vi "Word Report - Generate from Template.vi"() -> ()   [LabVIEW 2023]
doc: "This example shows how to generate a report from a Word document template. The template contains a preformatted table and a preformatted graph which are updated with Append Table to Report.vi and Excel Update Graph.vi."
uses:
  <vilib>/Utility/NIReport.llb/Report Type.ctl
  <vilib>/Utility/NIReport.llb/Append Report Text (str wrap).vi
  <vilib>/addons/_office/word.llb/Word Edit Cell ([str]).vi
  <vilib>/Utility/NIReport.llb/NI_report.lvclass
  <vilib>/addons/_office/NI_ReportGenerationToolkit.lvlib
  <vilib>/Utility/NIReport.llb/Word/NI_Word.lvclass
  <vilib>/Utility/NIReport.llb/NI_ReportGenerationCore.lvlib
panel:
  in  "Express VI?":bool
  in  "Test operator":string="Operator's name"
  in  "Pressure":string="100"
  in  "Humidity":string="70"
  in  "Temperature":string="20"
  in  "Data":string[][](table)=[["100", "41.7", "38.5"], ["125", "41.7", "35.2"], ["160", "41.5", "37.5"], ["200", "42.3", "42.5"], ["250", "46.9", "46.8"], ["315", "51.9", "52.6"], ["400", "52.3", "46.7"], ["500  ", "46.5", "41.6"], ["630", "42.3", "35.9"], ["800", "41.1", "32.6"]]
  # "Overview: This example shows how to generate a report from a template using either \nthe Word Report Generation VIs or the MS Office Report Express VI.\nRequirements: Report Generation Toolkit, Microsoft Word\nInstructions:\nRun the VI."
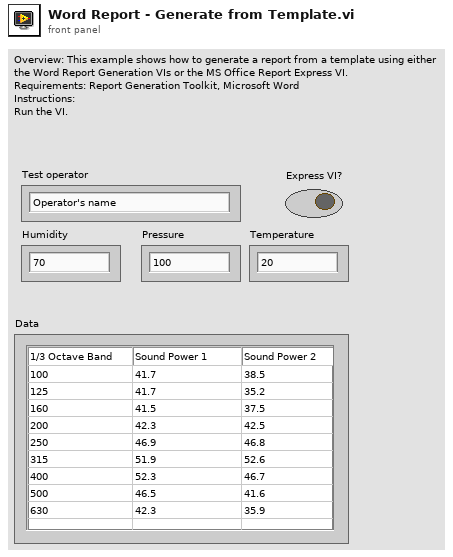
[diagram p1: front panel]
types:
  T1 = typedef "NI_ReportGenerationCore.lvlib/Report Type.ctl" = enum16{"HTML", "Word", "Excel"}
  T2 = cluster{"position (Excel)":cluster{"row":i32, "column":i32}, "name (Excel)":string, "bookmark (Word)":string}
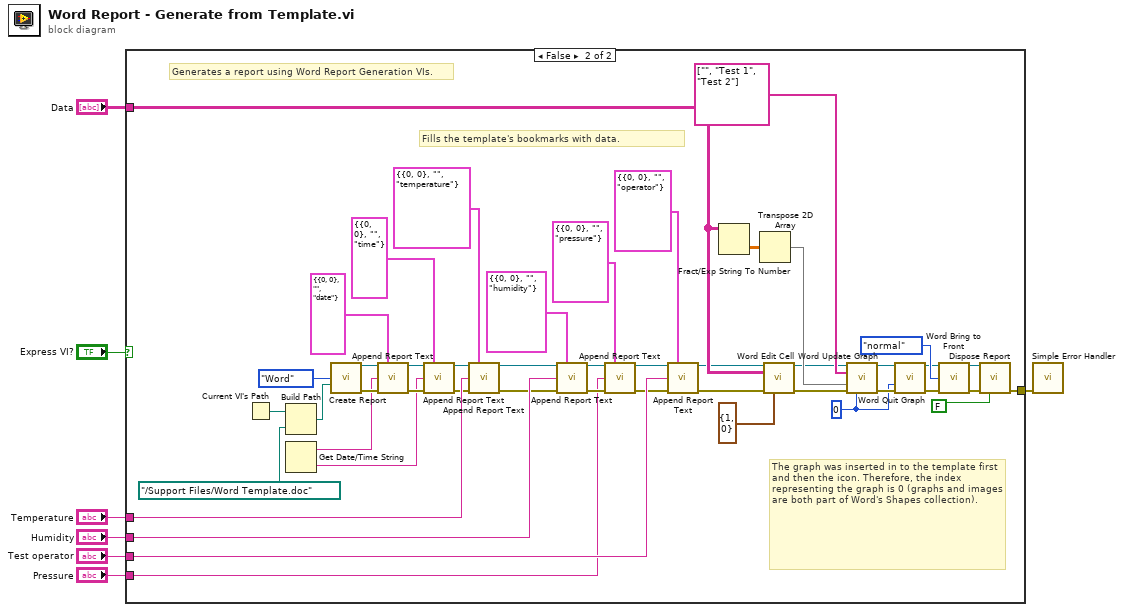
[diagram p0: block diagram]
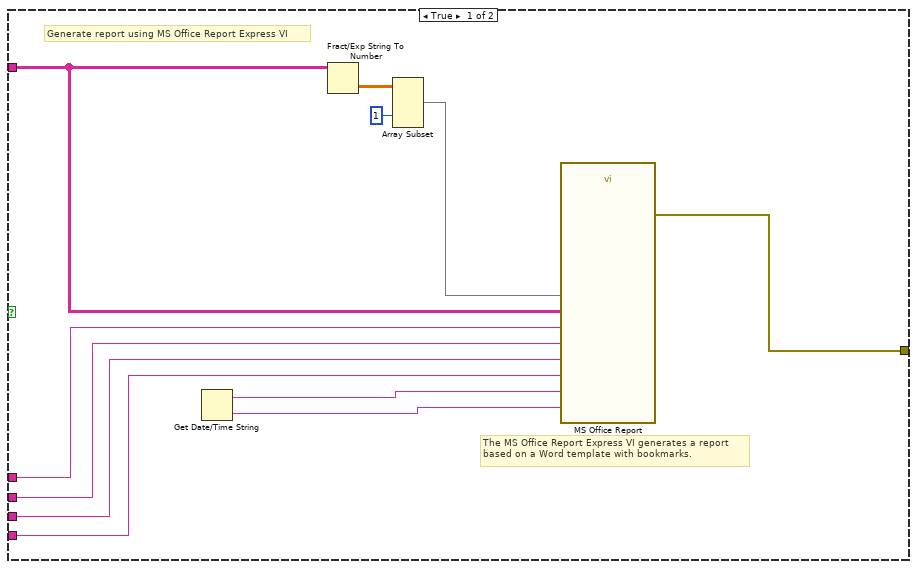
[diagram p2: hidden frame]
diagram:
  n1 = case shown="False" "Express VI?" {
    tunnel: "Temperature" -> [w10 w65]
    tunnel: "Humidity" -> [w15 w64]
    tunnel: "Test operator" -> [w12 w63]
    tunnel: "Data" -> [w14 w62]
    tunnel: [w13 w22] -> w2
    tunnel: "Pressure" -> [w11 w20]
    frame True {
      # "Generate report using MS Office Report Express VI"
      # "The MS Office Report Express VI generates a report\nbased on a Word template with bookmarks."
      n2 = Get Date/Time String() -> (date string=w9:string, time string=w8:string)  [unwired: 3 in]
      n3 = Fract/Exp String To Number(string=w14) -> (number=w18:dbl[][])  [unwired: 3 in, 1 out]
      n4 = Array Subset(array=w18, index (col)=1 ("index")) -> (w16:dbl[][])  [unwired: 3 in]
      n5 = call "MS Office Report"("chart"=w16, "data"=w14, "date"=w9, "humidity"=w15, "operator"=w12, "pressure"=w11, "temperature"=w10, "time"=w8) -> ("error out"=w13:errorcluster)  [unwired: 19 in]
    }
    frame False {
      w38 = i16 0 ("graph index")
      # "Fills the template's bookmarks with data."
      # "The graph was inserted in to the template first and then the icon. Therefore, the index representing the graph is 0 (graphs and images are both part of Word's Shapes collection)."
      # "Generates a report using Word Report Generation VIs."
      n6 = Current VI's Path() -> (path=w23:path)
      n7 = Build Path(base path=w23, name or relative path=path "../Support Files/Word Template.doc") -> (appended path=w26:path)
      n8 = Get Date/Time String() -> (date string=w24:string, time string=w25:string)  [unwired: 3 in]
      n9 = call <vilib>:"Create Report.vi"("report type"=Report_Type."Word" ("Report Type"), "template (empty)"=w26) -> ("report out"=w54:refnum<class "NI_report.lvclass">, "error out"=w60:errorcluster)  [unwired: 12 in]
      n10 = call-poly <vilib>:"Append Report Text.vi"("report in"=w54, "MS Office parameters"=T2 {"position (Excel)"={"row"=0, "column"=0}, "name (Excel)"="", "bookmark (Word)"="date"}, "text"=w24, "error in (no error)"=w60) -> ("report out"=w53:refnum<class "NI_report.lvclass">, "error out"=w59:errorcluster)  [unwired: 8 in, 2 out]
      n11 = call-poly <vilib>:"Append Report Text.vi"("report in"=w53, "MS Office parameters"=T2 {"position (Excel)"={"row"=0, "column"=0}, "name (Excel)"="", "bookmark (Word)"="time"}, "text"=w25, "error in (no error)"=w59) -> ("report out"=w52:refnum<class "NI_report.lvclass">, "error out"=w58:errorcluster)  [unwired: 8 in, 2 out]
      n12 = call-poly <vilib>:"Append Report Text.vi"("report in"=w52, "MS Office parameters"=T2 {"position (Excel)"={"row"=0, "column"=0}, "name (Excel)"="", "bookmark (Word)"="temperature"}, "text"=w65, "error in (no error)"=w58) -> ("report out"=w51:refnum<class "NI_report.lvclass">, "error out"=w57:errorcluster)  [unwired: 8 in, 2 out]
      n13 = call-poly <vilib>:"Append Report Text.vi"("report in"=w51, "MS Office parameters"=T2 {"position (Excel)"={"row"=0, "column"=0}, "name (Excel)"="", "bookmark (Word)"="humidity"}, "text"=w64, "error in (no error)"=w57) -> ("report out"=w50:refnum<class "NI_report.lvclass">, "error out"=w56:errorcluster)  [unwired: 8 in, 2 out]
      n14 = call-poly <vilib>:"Append Report Text.vi"("report in"=w50, "MS Office parameters"=T2 {"position (Excel)"={"row"=0, "column"=0}, "name (Excel)"="", "bookmark (Word)"="pressure"}, "text"=w20, "error in (no error)"=w56) -> ("report out"=w49:refnum<class "NI_report.lvclass">, "error out"=w55:errorcluster)  [unwired: 8 in, 2 out]
      n15 = call-poly <vilib>:"Append Report Text.vi"("report in"=w49, "MS Office parameters"=T2 {"position (Excel)"={"row"=0, "column"=0}, "name (Excel)"="", "bookmark (Word)"="operator"}, "text"=w63, "error in (no error)"=w55) -> ("report out"=w31:refnum<class "NI_report.lvclass">, "error out"=w29:errorcluster)  [unwired: 8 in, 2 out]
      n16 = Fract/Exp String To Number(string=w62) -> (number=w61:dbl[][])  [unwired: 3 in, 1 out]
      n17 = Transpose 2D Array(2D array=w61) -> (transposed array=w42:dbl[][])
      n18 = call-poly <vilib>:"Word Edit Cell.vi"("report in"=w31, "value"=w62, "error in (no error)"=w29, "start (0, 0)"=cluster{"row":i32, "column":i32} {"row"=1, "column"=0}) -> ("report out"=w30:refnum<class "NI_report.lvclass">, "error out"=w28:errorcluster)  [unwired: 10 in]
      n19 = call <vilib>:"Word Update Graph.vi"("report in"=w30, "row header"=string[] ["", "Test 1", "Test 2"], "graph data"=w42, "error in (no error)"=w28, "graph index (-1)"=w38) -> ("report out"=w40:refnum<class "NI_report.lvclass">, "error out"=w39:errorcluster)  [unwired: 9 in]
      n20 = call <vilib>:"Word Quit Graph.vi"("report in"=w40, "graph index (-1)"=w38, "error in (no error)"=w39) -> ("report out"=w35:refnum<class "NI_report.lvclass">, "error out"=w36:errorcluster)  [unwired: 11 in]
      n21 = call <vilib>:"Word Bring to Front.vi"("report in"=w35, "window state (maximized)"=enum16{"maximized", "minimized", "normal"}."normal", "error in (no error)"=w36) -> ("report out"=w33:refnum<class "NI_report.lvclass">, "error out"=w34:errorcluster)  [unwired: 11 in]
      n22 = call-dynamic "Dispose Report.vi"("report in"=w33, "error in (no error)"=w34, "close report? (T)"=FALSE ("Close Report? (T)")) -> ("error out"=w22:errorcluster)  [unwired: 12 in]
    }
  }
  n23 = call <vilib>:"Simple Error Handler.vi"("error in (no error)"=w2) -> ()  [unwired: 4 in, 5 out]
